vi "get Primary key.vi"(11 "Module Number":dbl=1.0) -> (3 "Primery Key":string[](array[string]))   [LabVIEW 2015, in "Copy of Untitled Library 1.lvlib"]
uses:
  Copy of Untitled Library 1.lvlib
  Controls/Enum Constant.ctl
panel:
  in  "error out 2":errorcluster
  out "error out":errorcluster
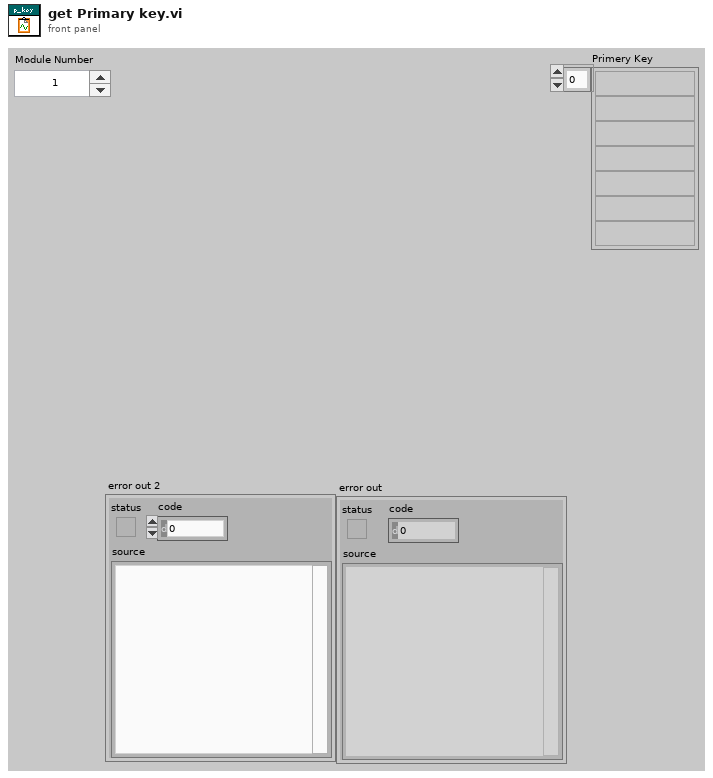
[diagram p1: front panel]
types:
  T1 = typedef "Enum Constant.ctl" = enum16{"Init", "Read", "Write"}
  T2 = typedef "FGV Data.ctl" = T3[]
  T3 = typedef "FGV Cluster Data.ctl" = cluster{"Manual/Automatic":bool, "UI Controllers ":string[], "UI Primery Key ":dbl[], "Caller Queue & MSG":T4, "Module ID":dbl, "DB Reference In":T5, "Products Columns":string[], "Cluster":cluster{"Delete Product":enum8{"Enabled", "Disabled", "Disabled and Grayed Out"}, "Add Product ":enum8{"Enabled", "Disabled", "Disabled and Grayed Out"}, "EDIT BATCH":enum8{"Enabled", "Disabled", "Disabled and Grayed Out"}, "Open Batch ":enum8{"Enabled", "Disabled", "Disabled and Grayed Out"}, "Close Batch":enum8{"Enabled", "Disabled", "Disabled and Grayed Out"}, "Delete Batch":enum8{"Enabled", "Disabled", "Disabled and Grayed Out"}, "Add Batch ":enum8{"Enabled", "Disabled", "Disabled and Grayed Out"}}}
  T4 = typedef "Queue and Caller MSG.ctl" = cluster{"Caller Queue":refnum<queue>, "Caller MSG":string}
  T5 = typedef "NI_Database_API.lvlib/Conn ObjectReference.ctl" = refnum<k1>
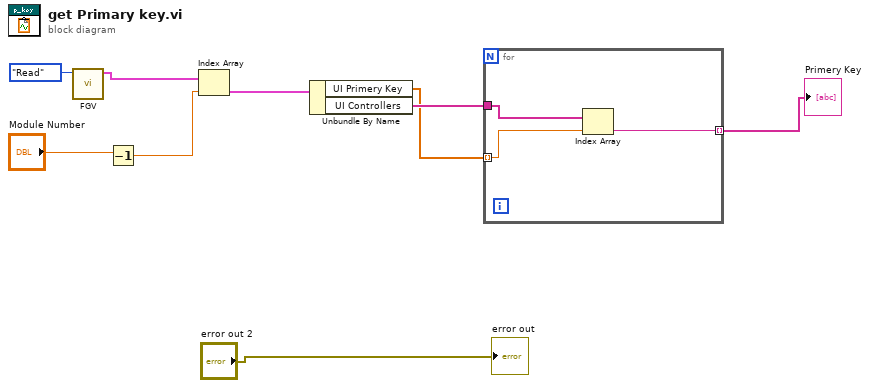
[diagram p0: block diagram]
diagram:
  n1 = call "FGV.vi"("Enum"=Enum_Constant."Read") -> ("Read Data"=w8:T2)  [unwired: 9 in, 1 out]
  n2 = Decrement(x="Module Number") -> (x-1=w1:dbl)
  n3 = Index Array(array=w8, index=w1) -> (element=w7:T3)
  n4 = Unbundle By Name(w7) -> ("UI Primery Key"=w5:dbl[], "UI Controllers"=w6:string[])
  n5 = for {
    tunnel: w6 -> [w11]
    tunnel: w5 -> [w12] mode=indexing
    tunnel: [w10] -> w4 mode=indexing
    n6 = Index Array(array=w11, index=w12) -> (element=w10:string)
  }
  "Primery Key" <- w4
  "error out" <- "error out 2"
